vi "Ultramat 23 Get Data.vi"(0 "VISA resource name":refnum<visa-resource-name>="OXYMAT", 5 "Source Address":u8=208 format="%.0x", 7 "Target Address":u8=16 format="%.0x", 9 "Gas selected":string, 11 "error in (no error)":errorcluster) -> (4 "VISA Session Out":refnum<visa-resource-name>, 6 "Message Header":T1 {"Source Address" format="%.0x"; "Target Address" format="%.0x"}, 8 "Data Array":string[][](array[string]), 14 "Success":bool, 15 "error out":errorcluster)   [LabVIEW 2020]
uses:
  instr.lib/Siemens ELAN/Message Header.ctl
  instr.lib/Siemens ELAN/Channel Status.ctl
  instr.lib/Siemens ELAN/Siemens ELAN.lvlib
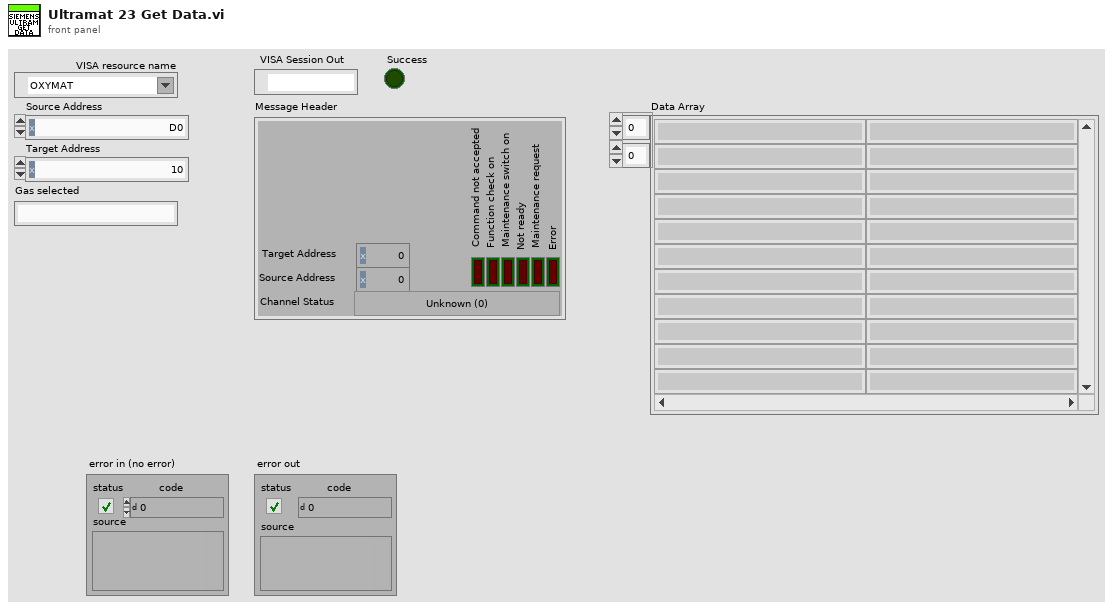
[diagram p1: front panel]
types:
  T1 = typedef "Siemens ELAN.lvlib/Message Header.ctl" = cluster{"Target Address":u8, "Source Address":u8, "Error":bool, "Maintenance request":bool, "Not ready":bool, "Maintenance switch on":bool, "Function check on":bool, "Command not accepted":bool, "Channel Status":T2}
  T2 = typedef "Siemens ELAN.lvlib/Channel Status.ctl" = enum8{"Unknown (0)", "Warm-up", "Pause", "Standby", "Measure", "Zero calibration", "Adjust component slope", "Unknown (7)", "Adjust curve dip", "Adjust linearization sensitivity", "Adjust temperature compensation", "Adjust pressure compensation", "Adjust linearization zero", "Adjust flow sensor", "Autocal", "Adjust phase", "Zero calibration of O2 sensor", "Synchronous zero calibration", "Purging for synchronous zero calibration", "Adjust analog output", "Adjust analog input", "Cleaning", "Unknown (>21)"}
  T3 = typedef "Siemens ELAN.lvlib/Unit Dimensions.ctl" = enum8{"Unknown (0)", "Pure number", "ppm", "ppb", "vpm", "vpm C1", "vpm C3", "vpm C6", "mg C/m^3", "mg/m^3", "%", "% v/v", "% of range", "% saturation", "%/°C", "%/K", "% w/w", "mV/pH", "mV/mbar", "nA/mbar", "S/m", "S/cm", "mS/m", "mS/cm", "uS/m", "uS/cm", "s", "min", "hr", "pA", "mA", "uV", "mV", "V", "mbar", "hPa", "ml/min", "kohm", "MOhm", "S", "°C", "Hz", "pH", "ug/l", "mg/l", "l/min", "uA", "mg/dm^3", "kPa", "kohm*cm", "MOhm*cm", "°", "Unknown (>51)"}
  T4 = typedef "Siemens ELAN.lvlib/Measured variables.ctl" = enum8{"Unknown (0)", "No component", "CO", "CO2", "CH4", "C6H14", "SO2", "NO", "NO2", "CHClF2 (R22)", "C3H8", "C4H10", "O2", "C5H12", "HC", "Pressure", "pH", "Temperature", "C2H4", "C2H2", "C3H6", "C4H6", "C4H8", "C2H6", "NH3", "N2O", "C6H6", "SF6", "CH3OH", "C2H5OH", "CH2Cl2", "C2H4Cl2", "CH3Cl", "C2H4O", "H2O (vapor)", "G/l", "Unknown (36)", "Unknown (37)", "Unknown (38)", "Unknown (39)", "Unknown (40)", "Unknown (41)", "Unknown (42)", "Unknown (43)", "Unknown (44)", "Unknown (45)", "Unknown (46)", "Unknown (47)", "Unknown (48)", "Unknown (49)", "Unknown (50)", "Unknown (51)", "Unknown (52)", "Unknown (53)", "Unknown (54)", "Unknown (55)", "Unknown (56)", "Unknown (57)", "Unknown (58)", "Unknown (59)", "Unknown (60)", "Unknown (61)", "Unknown (62)", "Unknown (63)", "Unknown (64)", "Unknown (65)", "Unknown (66)", "Unknown (67)", "Unknown (68)", "Unknown (69)", "Unknown (70)", "Unknown (71)", "Unknown (72)", "Unknown (73)", "Unknown (74)", "Unknown (75)", "Unknown (76)", "Unknown (77)", "Unknown (78)", "Unknown (79)", "Unknown (80)", "Unknown (81)", "Unknown (82)", "Unknown (83)", "Unknown (84)", "Unknown (85)", "Unknown (86)", "Unknown (87)", "Unknown (88)", "Unknown (89)", "Unknown (90)", "Unknown (91)", "Unknown (92)", "Unknown (93)", "Unknown (94)", "Unknown (95)", "Unknown ((96)", "Unknown (97)", "Unknown (98)", "Unknown (99)", "Ambient Pressure", "Unknown (>100)"}
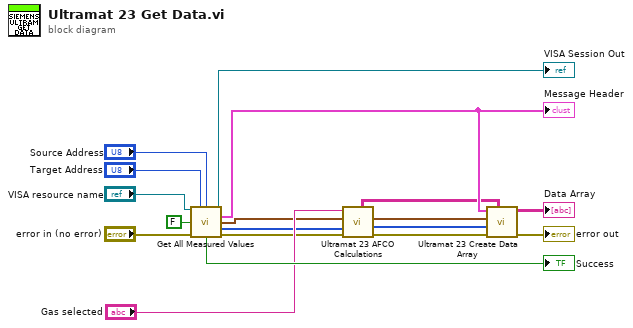
[diagram p0: block diagram]
diagram:
  n1 = call "Get All Measured Values.vi"("VISA Session In"="VISA resource name", "Target Address"="Target Address", "Source Address"="Source Address", "Use Broadcast?(F)"=FALSE, "error in (no error)"="error in (no error)") -> ("VISA Session Out"=→"VISA Session Out":refnum<visa-resource-name>, "Message Header"=w9:T1, "Measurements"=w7:cluster{"Measured value":dbl, "Dimension":T3}[], "Measured variables"=w6:T4[], "Success"=→"Success":bool, "error out"=w2:errorcluster)  [unwired: 5 in]
  "Message Header" <- w9
  n2 = call "Ultramat 23 AFCO Calculations.vi"("error in (no error)"=w2, "Measured variables"=w6, "Measurements"=w7, "Gas selected"="Gas selected") -> ("error out"=w3:errorcluster, "Measured variables Output"=w4:T4[], "Measurements Output"=w5:cluster{"Measured value":dbl, "Dimension":T3}[], "AFCO Data"=w1:string[][])  [unwired: 4 in]
  n3 = call "Ultramat 23 Create Data Array.vi"("AFCO Data"=w1, "error in (no error)"=w3, "Measured variables"=w4, "Measurements"=w5, "Message Header"=w9) -> ("error out"=→"error out":errorcluster, "Data Array"=→"Data Array":string[][])  [unwired: 5 in]
